vi "Evaluate Mood.vi"(7 "Mood Override Counter":u32, 8 "Override Mood":string, 9 "Cleanliness":i16=100, 10 "Hunger":i16, 11 "Energy":i16=100) -> (1 "Mood Override":string, 2 "Mood":string, 3 "Mood Override Counter out":u32)   [LabVIEW 2026]
uses:
  <vilib>/Analysis/NI_AAL_Polynomial.lvlib
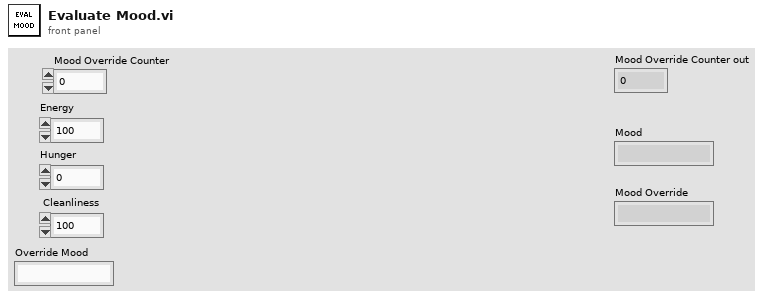
[diagram p1: front panel]
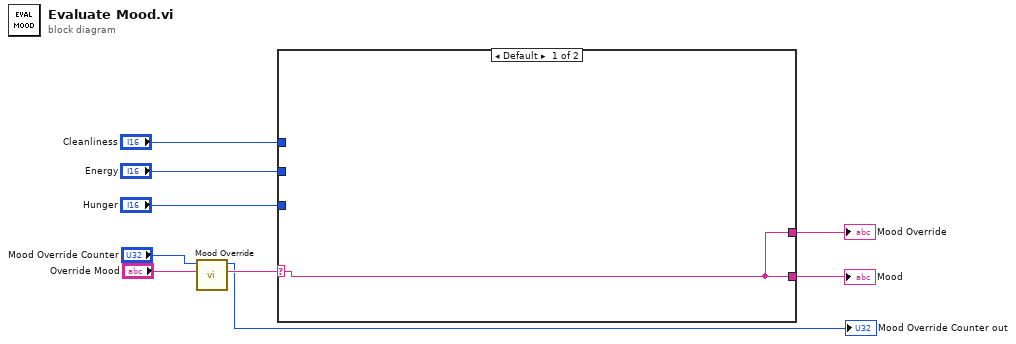
[diagram p0: block diagram]
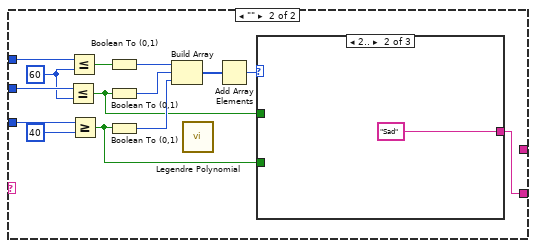
[diagram p2: hidden frame]
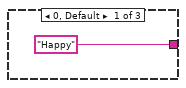
[diagram p3: hidden frame]
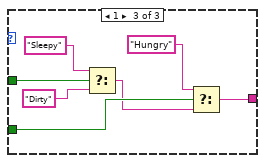
[diagram p4: hidden frame]
diagram:
  n1 = call "Mood Override.vi"("Mood Override in"="Override Mood", "Mood Override Counter in"="Mood Override Counter") -> ("Mood Override out"=w4:string, "Mood Override Counter out"=→"Mood Override Counter out":u32)  [unwired: 8 in]
  n2 = case shown="Default" w4 {
    selector: w4 -> [w10 _]
    tunnel: [w10 w13] -> w6
    tunnel: "Cleanliness" -> [_ w24]
    tunnel: "Energy" -> [_ w23]
    tunnel: "Hunger" -> [_ w21]
    tunnel: [w10 _] -> w1
    frame Default {
    }
    frame "" {
      w22 = i8 60 ("y")
      n3 = Less Or Equal?(x=w23, y=w22) -> (x <= y?=w11:bool)
      n4 = Less Or Equal?(x=w24, y=w22) -> (x <= y?=w19:bool)
      n5 = Greater Or Equal?(x=w21, y=i8 40) -> (x >= y?=w12:bool)
      n6 = Boolean To (0,1)(Boolean=w19) -> (0, 1=w18:i16)
      n7 = Boolean To (0,1)(Boolean=w11) -> (0, 1=w17:i16)
      n8 = Boolean To (0,1)(Boolean=w12) -> (0, 1=w16:i16)
      n9 = Build Array(w18, w17, w16) -> (w15:i16[])
      n10 = call <vilib>:"Legendre Polynomial.vi"() -> ()  [unwired: 10 in, 2 out]
      n11 = Add Array Elements(numeric array=w15) -> (sum=w14:i16)
      n12 = case shown="2.." w14 {
        tunnel: ["Happy" "Sad" w27] -> w13
        tunnel: w12 -> [_ _ w33]
        tunnel: w11 -> [_ _ w30]
        frame 0, Default {
        }
        frame 2.. {
        }
        frame 1 {
          n13 = Select(t="Sleepy", s=w30, f="Dirty") -> (s? t:f=w28:string)
          n14 = Select(t="Hungry", s=w33, f=w28) -> (s? t:f=w27:string)
        }
      }
    }
  }
  "Mood" <- w6
  "Mood Override" <- w1
